vi "IMAQ Get Pixel Value Wrapper.vi"(8 "Error In":errorcluster, 9 "Y Coordinate":i32, 10 "X Coordinate":i32, 11 "Image":T1) -> (0 "Error Out":errorcluster, 3 "Pixel Value":sgl, 4 "Point Outside Image":bool)   [LabVIEW 2021, in "Image.lvlib"]
uses:
  <vilib>/vision/Image Controls.llb/IMAQ Image.ctl
  Image.lvlib
  <vilib>/vision/NI_Vision_Development_Module.lvlib
  Time/Time.lvlib
panel:
  out "CPU (s)":dbl
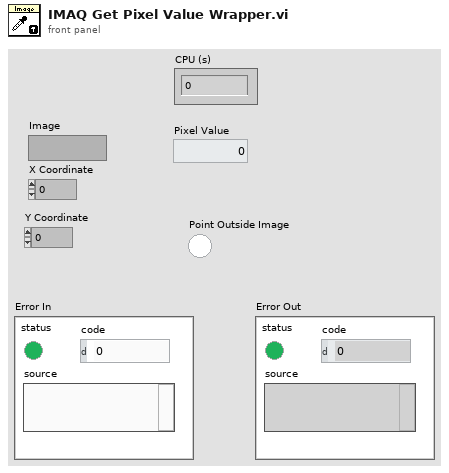
[diagram p1: front panel]
types:
  T1 = typedef "IMAQ Image.ctl" = refnum<image>
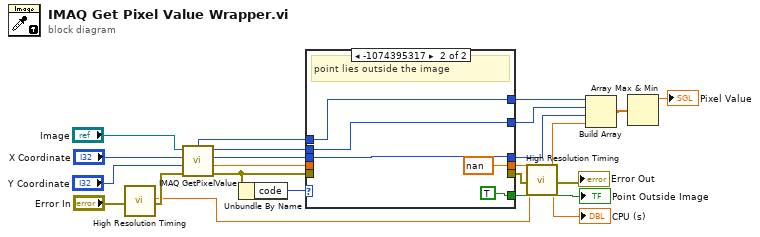
[diagram p0: block diagram]
diagram:
  n1 = call "High Resolution Timing.vi"("Error In"="Error In") -> ("elapsed (relative) seconds"=w8:dbl, "Error Out"=w10:errorcluster)  [unwired: 16 in, 1 out]
  n2 = call "IMAQ GetPixelValue"("Image"="Image", "X Coordinate"="X Coordinate", "Y Coordinate"="Y Coordinate", "error in (no error)"=w10) -> ("Pixel Value (U8)"=w12:u8, "Pixel Value (I16)"=w13:i16, "Pixel Value (U16)"=w11:u16, "Pixel Value (Float)"=w14:sgl, "error out"=w20:errorcluster)  [unwired: 2 in]
  n3 = Unbundle By Name(w20) -> ("code"=w21:i32)
  n4 = case shown="-1074395317" w21 {
    tunnel: w20 -> [w27 _]
    tunnel: [w27 _] -> w19
    tunnel: [_ TRUE ("Point Outside Image")] -> w15
    tunnel: w14 -> [w26 _]
    tunnel: [w26 sgl nan ("Pixel Value (Float)")] -> w3
    tunnel: w13 -> [w25 w28]
    tunnel: w12 -> [w24 w29]
    tunnel: w11 -> [w23 w30]
    tunnel: [w25 w28] -> w4
    tunnel: [w24 w29] -> w5
    tunnel: [w23 w30] -> w6
    frame 0, Default {
    }
    frame -1074395317 {
      # "point lies outside the image"
    }
  }
  "Point Outside Image" <- w15
  n5 = call "High Resolution Timing.vi"("relative seconds (NaN)"=w8, "Error In"=w19) -> ("elapsed (relative) seconds"=→"CPU (s)":dbl, "Error Out"=→"Error Out":errorcluster)  [unwired: 15 in, 1 out]
  n6 = Build Array(w6, w5, w4, w3) -> (w2:sgl[])
  n7 = Array Max & Min(array=w2) -> (max value=→"Pixel Value":sgl)  [unwired: 3 out]
